vi "GetTwoPointDis.vi"(1 "Point":cluster{"X":dbl, "Y":dbl}, 2 "Point 2":cluster{"X":dbl, "Y":dbl}) -> (0 "Dis":sgl)   [LabVIEW 2014]
uses:
  <vilib>/vision/NI_Vision_Development_Module.lvlib
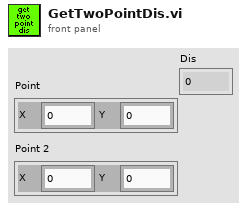
[diagram p1: front panel]
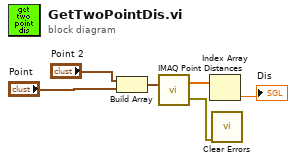
[diagram p0: block diagram]
diagram:
  n1 = Build Array("Point 2", "Point") -> (w5:cluster{"X":dbl, "Y":dbl}[])
  n2 = call "IMAQ Point Distances"("Points"=w5) -> ("Distances"=w6:sgl[], "error out"=w1:errorcluster)  [unwired: 4 in]
  n3 = Index Array(array=w6) -> (element=→"Dis":sgl)  [unwired: 1 in]
  n4 = call <vilib>:"Clear Errors.vi"("error in (no error)"=w1) -> ()  [unwired: 5 in, 2 out]
